vi "Prober_CloseSession.vi"(8 "error in (no error)":errorcluster, 11 "SemiProbe in":refnum<class "SemiProbe.lvclass">) -> (0 "error out":errorcluster, 3 "SemiProbe out":refnum<class "SemiProbe.lvclass">)   [LabVIEW 2019, in "SemiProbe.lvclass"]
uses:
  SemiProbe.lvclass
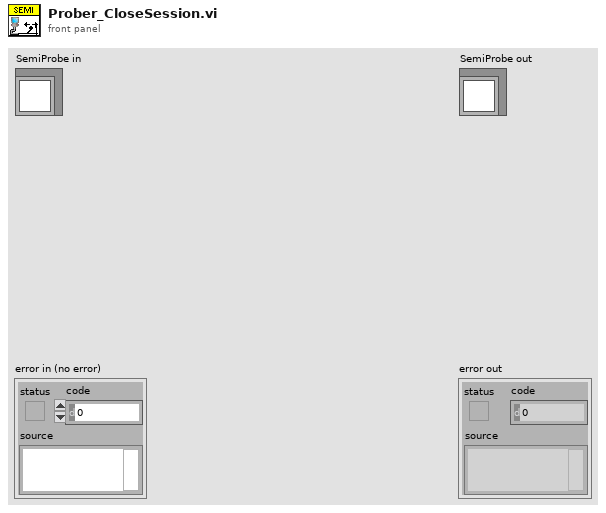
[diagram p1: front panel]
types:
  T1 = cluster{"address":string, "port":i32, "SP TCP Cnx ID":refnum<k5>, "mode (standard)":enum16{"Standard", "Buffered", "CRLF", "Immediate"}, "bytes to read":i32, "timeout (ms)":i32}
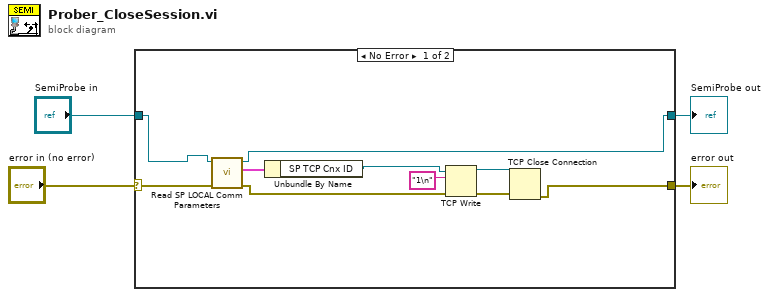
[diagram p0: block diagram]
diagram:
  n1 = case shown="No Error" "error in (no error)" {
    selector: "error in (no error)" -> [w11 w16]
    tunnel: [w5 w16] -> w3
    tunnel: "SemiProbe in" -> [w13 w15]
    tunnel: [w14 w15] -> w1
    frame No Error {
      n2 = call-dynamic "Read SP LOCAL Comm Parameters.vi"("error in (no error)"=w11, "SemiProbe in"=w13) -> ("error out"=w6:errorcluster, "SP LOCAL Comm Parameters"=w12:T1, "SemiProbe out"=w14:refnum<class "SemiProbe.lvclass">)  [unwired: 7 in]
      n3 = Unbundle By Name(w12) -> ("SP TCP Cnx ID"=w7:refnum<k5>)
      n4 = TCP Write(connection ID=w7, data in="1\n", error in (no error)=w6) -> (connection ID out=w9:refnum<k5>, error out=w10:errorcluster)  [unwired: 1 in, 1 out]
      n5 = TCP Close Connection(connection ID=w9, error in (no error)=w10) -> (error out=w5:errorcluster)  [unwired: 1 in, 1 out]
    }
    frame Error {
    }
  }
  "error out" <- w3
  "SemiProbe out" <- w1
